vi "Set ForceActuatorBoosterValveGainSettings.vi"(10 "ForceActuatorBoosterValveGainSettings":T1, 11 "Model in":refnum<class "Model.lvclass">) -> (3 "Model out":refnum<class "Model.lvclass">)   [LabVIEW 2016]
uses:
  Model.lvclass
  Typedefs/ForceActuatorBoosterValveGainSettings.ctl
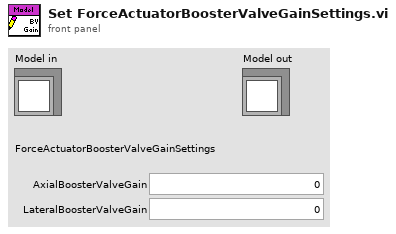
[diagram p1: front panel]
types:
  T1 = typedef "ForceActuatorBoosterValveGainSettings.ctl" = cluster{"AxialBoosterValveGain":sgl, "LateralBoosterValveGain":sgl}
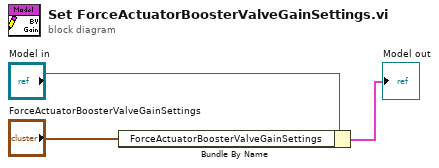
[diagram p0: block diagram]
diagram:
  n1 = Bundle By Name(cluster="Model in", "ForceActuatorBoosterValveGainSettings"="ForceActuatorBoosterValveGainSettings") -> (→"Model out":cluster{})
